vi "坐标旋转2D.vi"(8 "Error In":errorcluster caption="错误输入", 10 "dθ":dbl) -> (0 "Error Out":errorcluster caption="错误输出")   [LabVIEW 2012, in "几何工具.lvlib"]
uses:
  <vilib>/Utility/miscctls.llb/LVPointDoubleTypeDef.ctl
panel:
  out "输出点":T1[][](array[typedef])
  in  "输入点":T1[][](array[typedef])
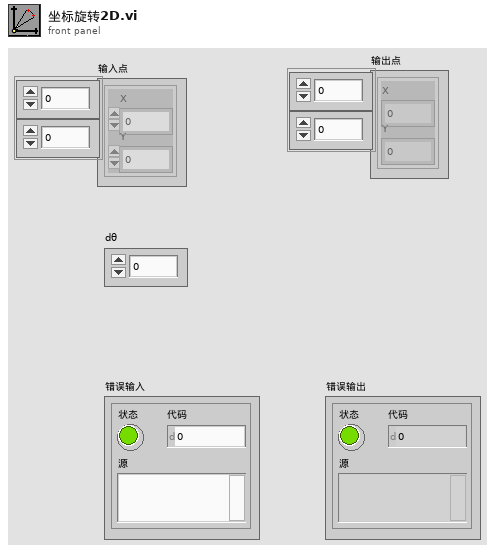
[diagram p1: front panel]
types:
  T1 = typedef "LVPointDoubleTypeDef.ctl" = cluster{"X":dbl, "Y":dbl}
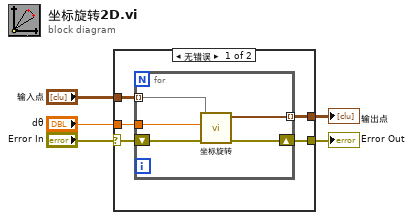
[diagram p0: block diagram]
diagram:
  n1 = case shown="无错误" "Error In" {
    selector: "Error In" -> [w8 w17]
    tunnel: [w7 w17] -> w4
    tunnel: "输入点" -> [w10 w16]
    tunnel: "dθ" -> [w6 _]
    tunnel: [w9 w16] -> w1
    frame No Error {
      n2 = for {
        tunnel: w10 -> [w15] mode=indexing
        tunnel: [w14] -> w9 mode=indexing
        shift-right: [w12] -> w7
        shift-left: w8 -> [w13]
        tunnel: w6 -> [w11]
        n3 = call-poly "坐标旋转.vi"("Error In"=w13, "dθ"=w11, "输入点"=w15) -> ("Error Out"=w12:errorcluster, "输出点"=w14:T1[])  [unwired: 7 in]
      }
    }
    frame Error {
    }
  }
  "Error Out" <- w4
  "输出点" <- w1
